vi "GenerateData.vi"(8 "error in (no error)":errorcluster, 11 "Stage_MadCityLab in":refnum<class "Stage_MadCityLab.lvclass">) -> (0 "error out":errorcluster, 2 "DataExchange":T1, 3 "Stage_MadCityLab out":refnum<class "Stage_MadCityLab.lvclass">)   [LabVIEW 2020, in "Stage_MadCityLab.lvlib" / "Stage_MadCityLab.lvclass"]
uses:
  Stage_MadCityLab.lvclass
  Hardware Abstraction Layer/Component/Device/Device/DataExchange.ctl
  Hardware Abstraction Layer/Component/Stage/Stage/Stage.lvclass
  Interface/DataListener/DataListener.lvclass
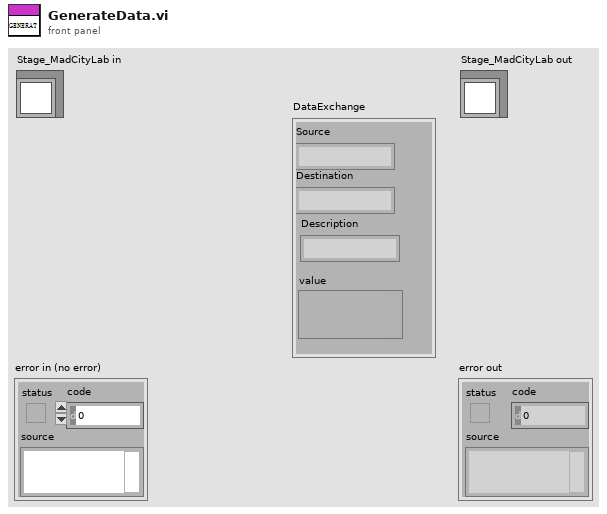
[diagram p1: front panel]
types:
  T1 = typedef "DataListener.lvclass/DataExchange.ctl" = cluster{"Source":string, "Destination":string, "Description":string, "value":variant}
  T2 = cluster{"Stage X Position":dbl, "Stage Y Position":dbl, "Stage Z Position":dbl}
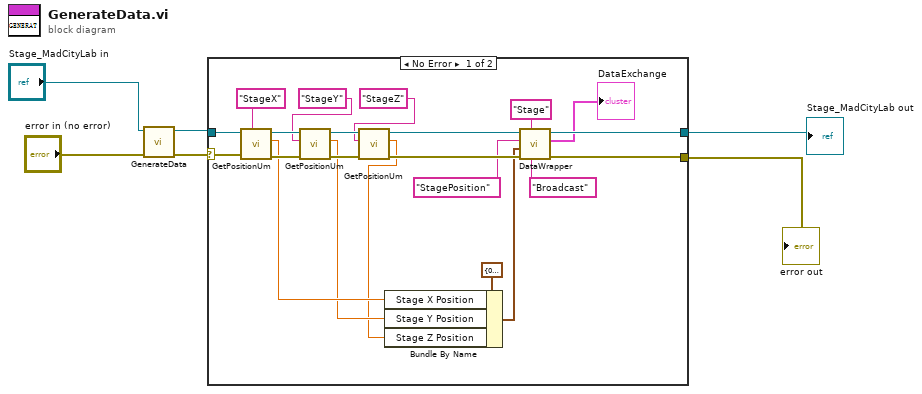
[diagram p0: block diagram]
diagram:
  n1 = call-parent "GenerateData.vi"("error in (no error)"="error in (no error)", "GRMActor in"="Stage_MadCityLab in") -> ("error out"=w3:errorcluster, "GRMActor out"=w4:refnum<class "Stage_MadCityLab.lvclass">)  [unwired: 7 in, 1 out]
  n2 = case shown="No Error" w3 {
    selector: w3 -> [w22 w30]
    tunnel: [w17 w30] -> w2
    tunnel: [w15 w29] -> w1
    tunnel: w4 -> [w28 w29]
    frame No Error {
      n3 = call-dynamic "GetPositionUm.vi"("error in (no error)"=w22, "Stage Label"="StageX", "Stage_MadCityLab in"=w28) -> ("error out"=w21:errorcluster, "Stage Position"=w9:dbl, "Stage_MadCityLab out"=w27:refnum<class "Stage_MadCityLab.lvclass">)  [unwired: 6 in]
      n4 = call-dynamic "GetPositionUm.vi"("error in (no error)"=w21, "Stage Label"="StageY", "Stage_MadCityLab in"=w27) -> ("error out"=w20:errorcluster, "Stage Position"=w8:dbl, "Stage_MadCityLab out"=w26:refnum<class "Stage_MadCityLab.lvclass">)  [unwired: 6 in]
      n5 = call-dynamic "GetPositionUm.vi"("error in (no error)"=w20, "Stage Label"="StageZ", "Stage_MadCityLab in"=w26) -> ("error out"=w19:errorcluster, "Stage Position"=w7:dbl, "Stage_MadCityLab out"=w16:refnum<class "Stage_MadCityLab.lvclass">)  [unwired: 6 in]
      n6 = Bundle By Name(cluster=T2 {"Stage X Position"=0.0, "Stage Y Position"=0.0, "Stage Z Position"=0.0} ("Cluster"), "Stage X Position"=w9, "Stage Y Position"=w8, "Stage Z Position"=w7) -> (w13:T2)
      n7 = call-dynamic "DataWrapper.vi"("Destination"="Broadcast" ("Type"), "Source"="Stage", "error in (no error)"=w19, "value"=w13, "Description"="StagePosition" ("Target"), "GRMActor in"=w16) -> ("error out"=w17:errorcluster, "DataExchange"=→"DataExchange":T1, "GRMActor out"=w15:refnum<class "Stage_MadCityLab.lvclass">)  [unwired: 3 in]
    }
    frame Error {
    }
  }
  "error out" <- w2
  "Stage_MadCityLab out" <- w1
